vi "set Player Positions.vi"(9 "Player 2 Position":T1, 10 "Player 1 Position":T1, 11 "Camera in":refnum<class "Camera.lvclass">) -> (3 "Camera out":refnum<class "Camera.lvclass">)   [LabVIEW 2018, in "Camera.lvclass"]
uses:
  Camera.lvclass
  LabSDL2/Source/Libraries/SDL2 Utility/Point (I32).ctl
  LabSDL2/Source/Libraries/SDL2 Utility/SDL2 Utility.lvlib
  Math/Math.lvlib
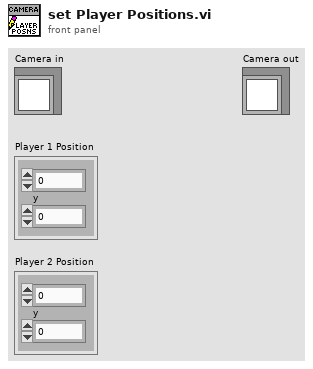
[diagram p1: front panel]
types:
  T1 = typedef "SDL2 Utility.lvlib/Point (I32).ctl" = cluster{"x":i32, "y":i32}
  T2 = typedef "Constants.ctl" = cluster{"Colours":cluster{"OK":u32, "Warning":u32, "Error":u32, "Red":u32, "Green":u32, "Blue":u32, "Yellow":u32}, "System":cluster{"Target Frames Second":dbl, "World Size":T1, "Window Size":T1, "Viewport Size":T1, "Sidebar Scaling":sgl, "Sidebar Width":i32, "SC2 Frame Rate [Seconds/Frame]":sgl}, "Game":cluster{"Maximum Asteroids":i32, "Max Energy":i32, "Max Crew":i32, "Maximum Stars":i32}}
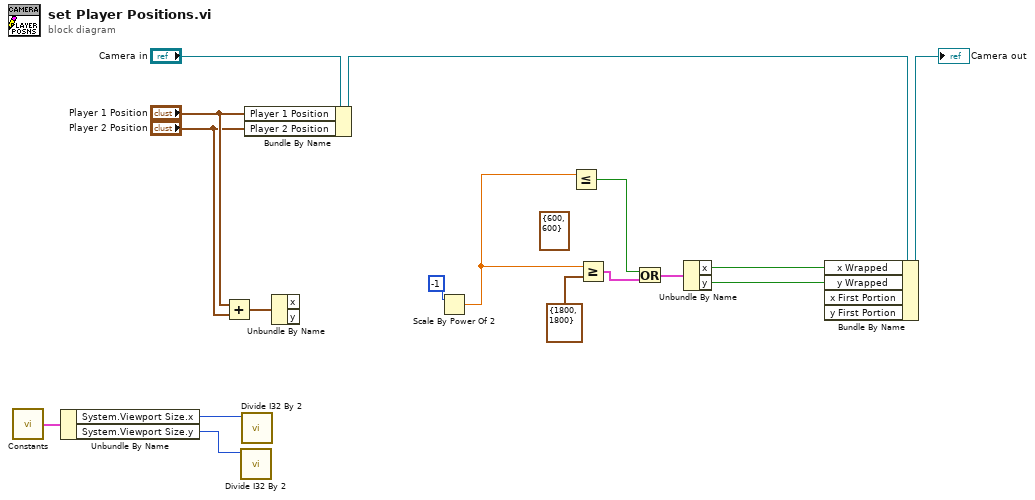
[diagram p0: block diagram]
diagram:
  (unwired) T1 {"x"=600, "y"=600} ("y")
  n1 = call "Constants.vi"() -> ("Constants"=w16:T2)
  n2 = Unbundle By Name(w16) -> ("System.Viewport Size.x"=w3:i32, "System.Viewport Size.y"=w2:i32)
  n3 = Add(x="Player 1 Position", y="Player 2 Position") -> (x+y=w1:T1)
  n4 = call "Divide I32 By 2.vi"("Value"=w2) -> ()  [unwired: 10 in, 1 out]
  n5 = call "Divide I32 By 2.vi"("Value"=w3) -> ()  [unwired: 10 in, 1 out]
  n6 = Bundle By Name(cluster="Camera in", "Player 1 Position"="Player 1 Position", "Player 2 Position"="Player 2 Position") -> (w13:refnum<class "Camera.lvclass">)
  n7 = Unbundle By Name(w1) -> ()  [unwired: 2 out]
  n8 = Scale By Power Of 2(n=i16 -1) -> (x*2^n=w5:ext)  [unwired: 1 in]
  n9 = Less Or Equal?(x=w5) -> (x <= y?=w4:bool)  [unwired: 1 in]
  n10 = Greater Or Equal?(x=w5, y=T1 {"x"=1800, "y"=1800}) -> (x >= y?=w8:cluster{"x":bool, "y":bool})
  n11 = Or(x=w4, y=w8) -> (x .or. y?=w7:cluster{"x":bool, "y":bool})
  n12 = Unbundle By Name(w7) -> ("x"=w10:bool, "y"=w12:bool)
  n13 = Bundle By Name(cluster=w13, "x Wrapped"=w10, "y Wrapped"=w12) -> (→"Camera out":refnum<class "Camera.lvclass">)  [unwired: 2 in]
